vi "Enable Channel(s) Output.vi"(8 "error in (no error)":errorcluster, 9 "Output (On = True)":bool, 10 "Channel(s)":i32[](array[numeric]), 11 "PXIe5413 in":refnum<class "PXIe5413.lvclass">) -> (0 "error out":errorcluster, 3 "PXIe5413 out":refnum<class "PXIe5413.lvclass">)   [LabVIEW 2018, in "PXIe5413.lvlib" / "PXIe5413.lvclass"]
uses:
  PXIe5413.lvclass
  PPLs/Function Generator/Parent/Function Generator.lvlibp/Function Generator.lvclass
  C:/Projects/LabVIEW/PPLs/Function Generator/Parent/Function Generator.lvlibp/Function Generator.lvclass
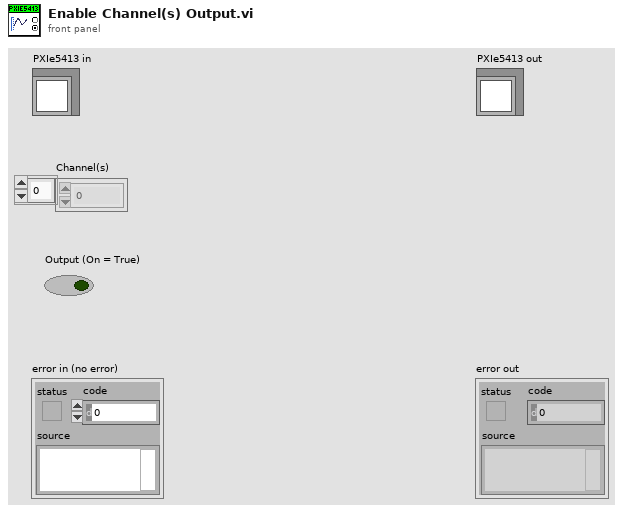
[diagram p1: front panel]
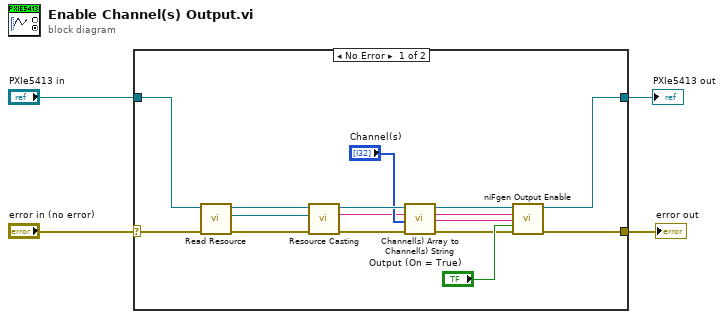
[diagram p0: block diagram]
diagram:
  n1 = case shown="No Error" "error in (no error)" {
    selector: "error in (no error)" -> [w18 w20]
    tunnel: [w6 w20] -> w3
    tunnel: [w7 w19] -> w2
    tunnel: "PXIe5413 in" -> [w17 w19]
    frame No Error {
      n2 = call "Read Resource.vi"("error in (no error)"=w18, "Function Generator in"=w17) -> ("error out"=w16:errorcluster, "Resource"=w5:refnum<visa-resource-name>, "Function Generator out"=w15:refnum<class "PXIe5413.lvclass">)  [unwired: 7 in]
      n3 = call "Resource Casting.vi"("error in (no error)"=w16, "VISA Resource In"=w5, "PXIe5413 in"=w15) -> ("error out"=w11:errorcluster, "Casted Resource"=w9:string, "PXIe5413 out"=w13:refnum<class "PXIe5413.lvclass">)  [unwired: 6 in]
      n4 = call "Channel(s) Array to Channel(s) String.vi"("error in (no error)"=w11, "Channel(s)"="Channel(s)", "PXIe5413 in"=w13) -> ("error out"=w10:errorcluster, "Channels String"=w8:string, "PXIe5413 out"=w7:refnum<class "PXIe5413.lvclass">)  [unwired: 6 in]
      n5 = call <instrlib>:"niFgen Output Enable.vi"("error in (no error)"=w10, "Output Enable (default: True)"="Output (On = True)", "Channel Name"=w8, "Instrument Handle"=w9) -> ("error out"=w6:errorcluster)  [unwired: 6 in, 1 out]
    }
    frame Error {
    }
  }
  "error out" <- w3
  "PXIe5413 out" <- w2
